vi "GetDataForExcel.ExtractActivity.vi"(7 "ReportSelection":u16, 8 "error in (no error)":errorcluster, 9 "Active":string[](array[string]), 10 "Normal":string[](array[string]), 11 "path in":path) -> (0 "error out":errorcluster, 2 "Data":dbl[][](array[numeric]), 3 "Names":string[](array[string]))   [LabVIEW 2013, in "main.lvlib"]
uses:
  main.lvlib
  <userlib>/_OpenG.lib/array/array.llb/Filter 1D Array with Scalar (String)__ogtk.vi
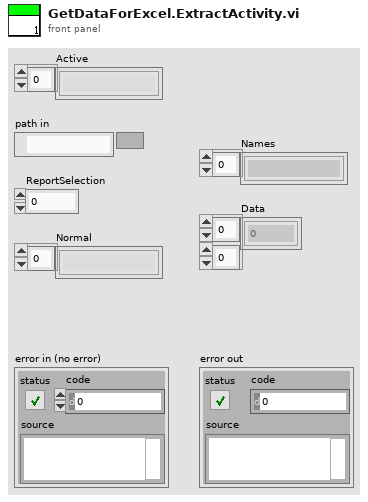
[diagram p1: front panel]
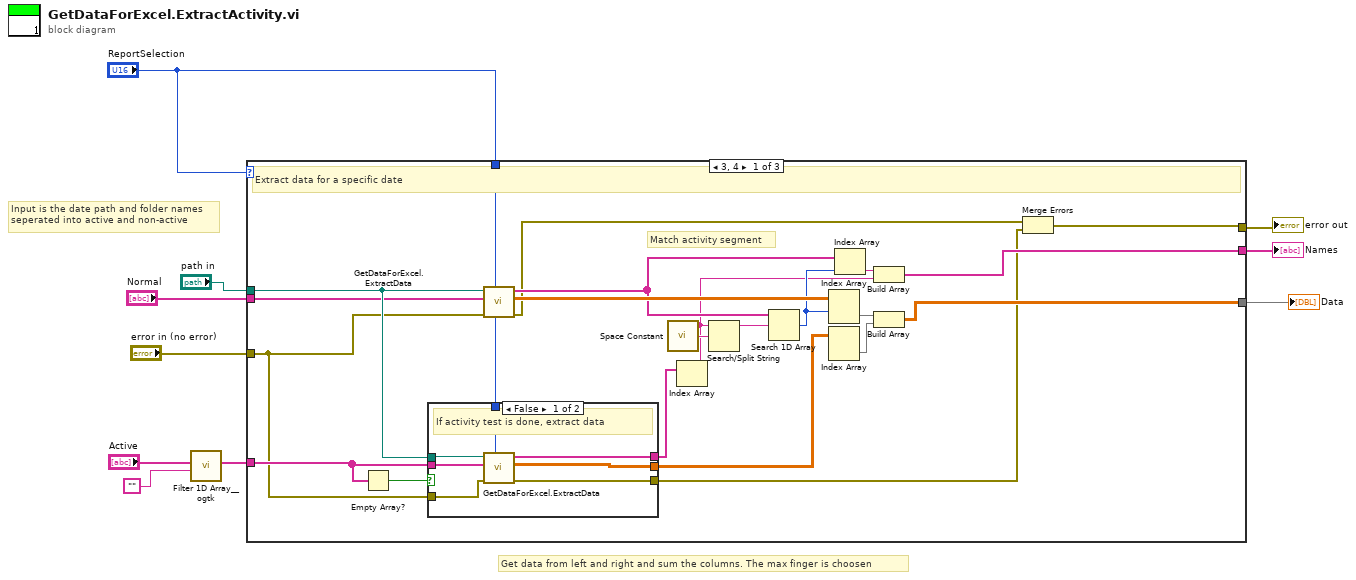
[diagram p0: block diagram]
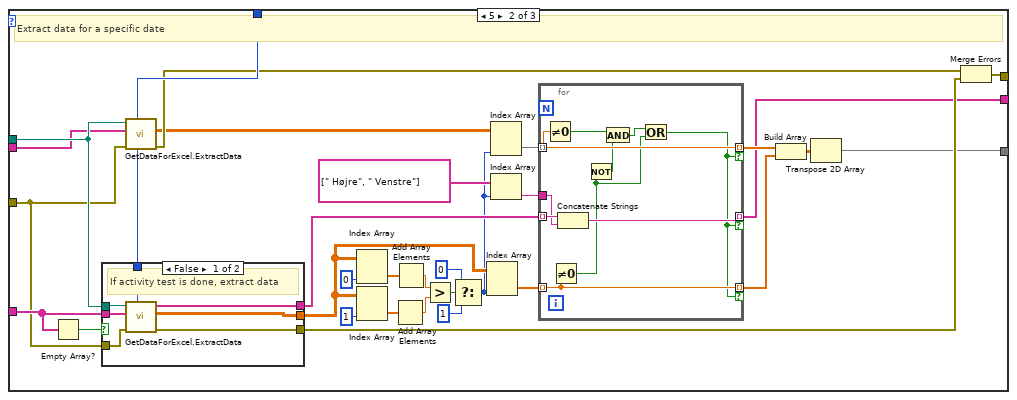
[diagram p3: hidden frame]
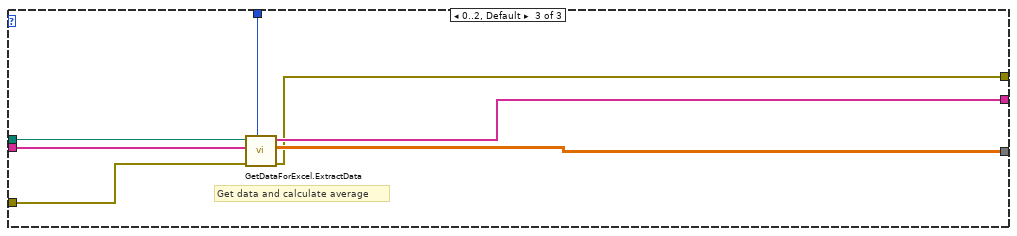
[diagram p5: hidden frame]
diagram:
  # "Get data from left and right and sum the columns. The max finger is choosen"
  # "Input is the date path and folder names\nseperated into active and non-active"
  n1 = call-poly <userlib>:"Filter 1D Array__ogtk.vi"("items to filter"="", "array"="Active") -> ("filtered array"=w1:string[])  [unwired: 4 in, 1 out]
  n2 = case shown="3, 4" "ReportSelection" {
    tunnel: [w22 w44 w96] -> w10
    tunnel: [w21 w46 w95] -> w9
    tunnel: "ReportSelection" -> [w32 w71 w94]
    tunnel: "path in" -> [w31 w70 w93]
    tunnel: w1 -> [w30 w69 _]
    tunnel: "Normal" -> [w28 w67 w92]
    tunnel: "error in (no error)" -> [w12 w64 w91]
    tunnel: [w14 w66 w90] -> w4
    frame 3, 4 {
      # "Match activity segment"
      # "Extract data for a specific date"
      n3 = Empty Array?(array=w30) -> (empty?=w29:bool)
      n4 = case shown="False" w29 {
        tunnel: w30 -> [w39 _]
        tunnel: w31 -> [w38 _]
        tunnel: w32 -> [w37 _]
        tunnel: [w36 _] -> w27
        tunnel: [w35 _] -> w24
        tunnel: [w34 w40] -> w13
        tunnel: w12 -> [w33 w40]
        frame False {
          # "If activity test is done, extract data"
          n5 = call "GetDataForExcel.ExtractData.vi"("Report Type"=w37, "Error In"=w33, "Folders"=w39, "Path"=w38) -> ("Error Out"=w34:errorcluster, "Data"=w35:dbl[][], "Names"=w36:string[])  [unwired: 5 in]
        }
        frame True {
        }
      }
      n6 = call "GetDataForExcel.ExtractData.vi"("Report Type"=w32, "Error In"=w12, "Folders"=w28, "Path"=w31) -> ("Error Out"=w11:errorcluster, "Data"=w26:dbl[][], "Names"=w20:string[])  [unwired: 5 in]
      n7 = call <vilib>:"Space Constant.vi"() -> ("String"=w17:string)
      n8 = Index Array(array=w27) -> (element=w15:string)  [unwired: 1 in]
      n9 = Search/Split String(string=w15, search string/char (-)=w17) -> (substring before match=w16:string)  [unwired: 1 in, 2 out]
      n10 = Search 1D Array(1D array=w20, element=w16) -> (index of element=w19:i32)  [unwired: 1 in]
      n11 = Index Array(array=w26, index (row)=w19) -> (element=w25:dbl[])  [unwired: 1 in]
      n12 = Index Array(array=w24) -> (element=w23:dbl[])  [unwired: 2 in]
      n13 = Index Array(array=w20, index=w19) -> (element=w18:string)
      n14 = Build Array(w18, w15) -> (w21:string[])
      n15 = Build Array(w25, w23) -> (w22:dbl[][])
      n16 = Merge Errors(w11, w13) -> (w14:errorcluster)
    }
    frame 5 {
      # "Extract data for a specific date"
      n17 = Empty Array?(array=w69) -> (empty?=w68:bool)
      n18 = case shown="False" w68 {
        tunnel: w69 -> [w88 _]
        tunnel: w70 -> [w87 _]
        tunnel: w71 -> [w86 _]
        tunnel: [w85 _] -> w51
        tunnel: [w84 _] -> w53
        tunnel: [w83 w89] -> w65
        tunnel: w64 -> [w82 w89]
        frame False {
          # "If activity test is done, extract data"
          n19 = call "GetDataForExcel.ExtractData.vi"("Report Type"=w86, "Error In"=w82, "Folders"=w88, "Path"=w87) -> ("Error Out"=w83:errorcluster, "Data"=w84:dbl[][], "Names"=w85:string[])  [unwired: 5 in]
        }
        frame True {
        }
      }
      n20 = call "GetDataForExcel.ExtractData.vi"("Report Type"=w71, "Error In"=w64, "Folders"=w67, "Path"=w70) -> ("Error Out"=w63:errorcluster, "Data"=w50:dbl[][])  [unwired: 5 in, 1 out]
      n21 = Index Array(array=w53, index (col)=0 ("index")) -> (element=w62:dbl[])  [unwired: 1 in]
      n22 = Index Array(array=w53, index (col)=1 ("index")) -> (element=w54:dbl[])  [unwired: 1 in]
      n23 = Add Array Elements(numeric array=w54) -> (sum=w61:dbl)
      n24 = Add Array Elements(numeric array=w62) -> (sum=w59:dbl)
      n25 = Greater?(x=w59, y=w61) -> (0:w60:bool)
      n26 = Select(t=0, s=w60, f=1) -> (s? t:f=w42:i32)
      n27 = Index Array(array=w53, index (col)=w42) -> (element=w52:dbl[])  [unwired: 1 in]
      n28 = Index Array(array=w50, index (col)=w42) -> (element=w49:dbl[])  [unwired: 1 in]
      n29 = Index Array(array=string[] [" Højre", " Venstre"], index=w42) -> (element=w41:string)
      n30 = for {
        tunnel: w52 -> [w81] mode=indexing
        tunnel: w51 -> [w80] mode=indexing
        tunnel: w49 -> [w77] mode=indexing
        tunnel: [w77] -> w48 mode=indexing if=w72
        tunnel: [w79] -> w46 mode=indexing if=w72
        tunnel: [w81] -> w47 mode=indexing if=w72
        tunnel: w41 -> [w78]
        n31 = Not Equal To 0?(x=w77) -> (x != 0?=w75:bool)
        n32 = Not Equal To 0?(x=w81) -> (x != 0?=w73:bool)
        n33 = Concatenate Strings(w80, w78) -> (w79:string)
        n34 = Not(x=w73) -> (.not. x?=w76:bool)
        n35 = And(x=w75, y=w76) -> (x .and. y?=w74:bool)
        n36 = Or(x=w74, y=w73) -> (x .or. y?=w72:bool)
      }
      n37 = Build Array(w48, w47) -> (w45:dbl[][])
      n38 = Transpose 2D Array(2D array=w45) -> (transposed array=w44:dbl[][])
      n39 = Merge Errors(w63, w65) -> (w66:errorcluster)
    }
    frame 0..2, Default {
      # "Get data and calculate average"
      n40 = call "GetDataForExcel.ExtractData.vi"("Report Type"=w94, "Error In"=w91, "Folders"=w92, "Path"=w93) -> ("Error Out"=w90:errorcluster, "Data"=w96:dbl[][], "Names"=w95:string[])  [unwired: 5 in]
    }
  }
  "Data" <- w10
  "Names" <- w9
  "error out" <- w4
